vi "Write Path.vi"(8 "error in (no error)":errorcluster, 10 "Path":path, 11 "File in":refnum<class "File.lvclass">) -> (0 "error out":errorcluster, 3 "File out":refnum<class "File.lvclass">)   [LabVIEW 2014, in "LabVIEW Universal Transcriptor SD Card Library.lvlib" / "File.lvclass"]
uses:
  File.lvclass
  File.lvclass/File.ctl
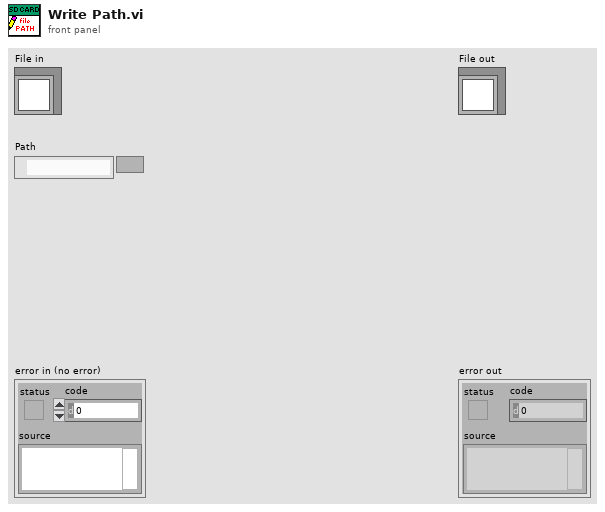
[diagram p1: front panel]
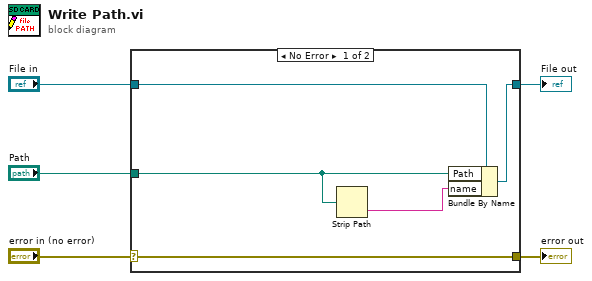
[diagram p0: block diagram]
diagram:
  n1 = case shown="No Error" "error in (no error)" {
    selector: "error in (no error)" -> [w10 w11]
    tunnel: [w10 w11] -> w4
    tunnel: [w8 w12] -> w2
    tunnel: "File in" -> [w9 w12]
    tunnel: "Path" -> [w7 _]
    frame No Error {
      n2 = Strip Path(path=w7) -> (name=w6:string)  [unwired: 1 out]
      n3 = Bundle By Name(cluster=w9, "Path"=w7, "name"=w6) -> (w8:refnum<class "File.lvclass">)
    }
    frame Error {
    }
  }
  "error out" <- w4
  "File out" <- w2
